vi "Initialise.vi"(8 "error in (no error)":errorcluster, 10 "Instrument Ref":string, 11 "NI DMM4072 in":refnum<class "NI DMM4072.lvclass">) -> (0 "error out":errorcluster, 3 "NI DMM4072 out":refnum<class "NI DMM4072.lvclass">)   [LabVIEW 2021, in "Concrete.lvlib" / "NI DMM4072.lvclass"]
uses:
  NI DMM4072.lvclass
  NI DMM4072.lvclass/NI DMM4072.ctl
  Harware Abstraction/MultiIO/MultiFunction IO.lvclass
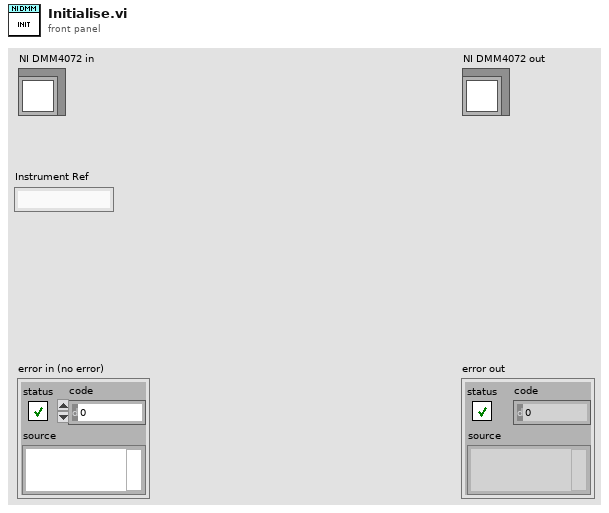
[diagram p1: front panel]
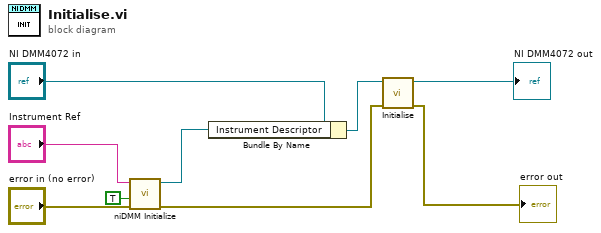
[diagram p0: block diagram]
diagram:
  n1 = call <instrlib>:"niDMM Initialize.vi"("error in (no error)"="error in (no error)", "Reset"=TRUE, "Instrument Descriptor"="Instrument Ref") -> ("instrument handle out"=w2:refnum<k15>)  [unwired: 7 in, 1 out]
  n2 = Bundle By Name(cluster="NI DMM4072 in", "Instrument Descriptor"=w2) -> (w3:refnum<class "NI DMM4072.lvclass">)
  n3 = call-parent "Initialise.vi"("error in (no error)"="error in (no error)", "Instrument in"=w3) -> ("error out"=→"error out":errorcluster, "Instrument out"=→"NI DMM4072 out":refnum<class "NI DMM4072.lvclass">)  [unwired: 8 in]
